vi "TRIG_CHAN_AUX_DEL.vi"(0 "VISA IN":refnum<visa-resource-name>, 1 "Aux":i32, 2 "Delay":dbl, 5 "error in":errorcluster, 7 "Channel":i32) -> (14 "VISA Out":refnum<visa-resource-name>, 19 "error out":errorcluster)   [LabVIEW 2018, in "PNA-X.lvlib"]
doc: "TRIGger:CHANnel<ch>:AUX<n>:DELay <num> \n(Read-Write) Specifies the delay that should be applied by the PNA after the Aux trigger input is \nreceived and before the acquisition is made. \nParameters \n<ch> Any existing channel number. If unspecified, value is set to 1. \n<n> Rear panel connectors used to send or receive signals. \nPNA-X - choose from 1 (AUX TRIG 1 IN) or 2 (AUX TRIG 2 IN) \nAll other models: choose 1. \nIf unspecified, value is set to 1. \n<num> Delay value in seconds. Choose a value between 0 and 3.0 seconds. \nExamples TRIG:CHAN:AUX:DEL .5 \ntrigger:channel2:aux2:delay 1.5 \nQuery Syntax TRIGger:CHANnel<ch>:AUX<n>:DELay? \nReturn Type Numeric \nDefault 0 \n1887"
uses:
  PNA-X.lvlib
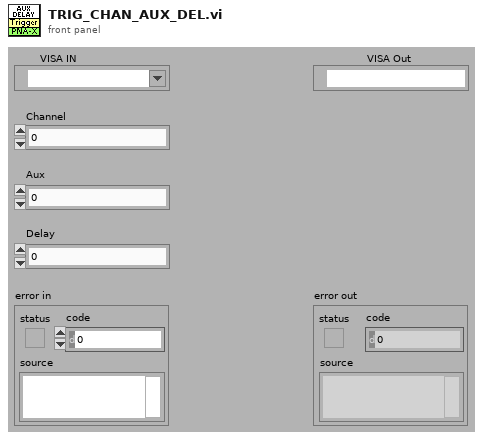
[diagram p1: front panel]
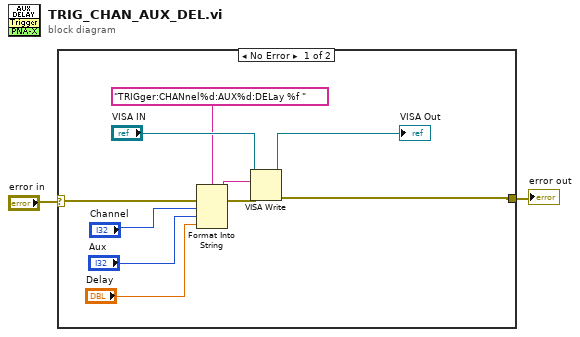
[diagram p0: block diagram]
diagram:
  n1 = case shown="No Error" "error in" {
    selector: "error in" -> [w12 w13]
    tunnel: [w8 w13] -> w1
    frame No Error {
      n2 = Format Into String(format string="TRIGger:CHANnel%d:AUX%d:DELay %f " ("Cmdline"), error in=w12, "Channel", "Aux", "Delay") -> (resulting string=w10:string, error out=w11:errorcluster)  [unwired: 1 in]
      n3 = VISA Write(VISA resource name="VISA IN", write buffer=w10, error in (no error)=w11) -> (VISA resource name out=→"VISA Out":refnum<visa-resource-name>, error out=w8:errorcluster)  [unwired: 1 out]
    }
    frame Error {
    }
  }
  "error out" <- w1
